vi "Host-Version-Top-Level.vi"() -> ()   [LabVIEW 2015]
uses:
  LabVIEW/SETI_LV/SETI_LV.lvlib
panel:
  out "Results Match":bool
  in  "error in":errorcluster
  in  "Run #\nto Load":i32=1
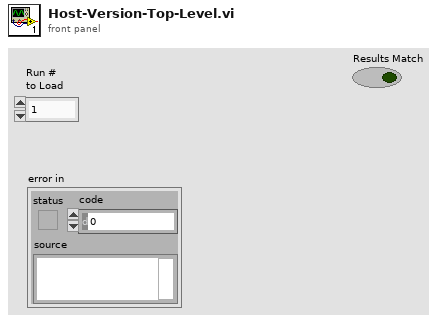
[diagram p1: front panel]
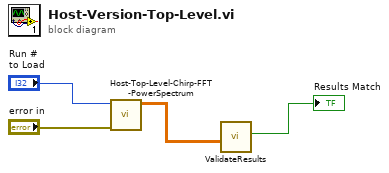
[diagram p0: block diagram]
diagram:
  n1 = call "Host-Top-Level-Chirp-FFT-PowerSpectrum.vi"("error in"="error in", "Run Number\nto Load"="Run #\nto Load") -> ("PowerSpectrum"=w2:dbl[][])  [unwired: 9 in]
  n2 = call "ValidateResults.vi"("Array in"=w2) -> ("Boolean"=→"Results Match":bool)  [unwired: 9 in, 1 out]
